vi "VI Properties - Front Panel States.vi"() -> ()   [LabVIEW 2019]
doc: "This VI demonstrates how to programmatically change the state of the front panel window. \n\nThere are six states that are related to the front panel of a VI; Standard, Maximize, Minimize, Hidden, Closed and Invalid. All states are read/write with the exception of Invalid, which is read only. The Standard state sets the VI to its default front panel state. The Maximize state will maximize the VI to full screen size. Minimize state is used to minimize the VI to the task bar. When using the Hidden state, the VI is still in memory, yet the front panel is hidden from view. The Closed state will also hide the front panel of the VI, but the front panel objects of the VI are no longer in memory. Lastly, the Invalid state is returned if an attempt is made to apply a window state at a time when it cannot be applied to the VI."
panel:
  in  "Stop":bool
  in  "Hidden":bool
  in  "Standard":bool
  in  "Minimize":bool
  in  "Maximize":bool
  # "Overview: Programmatically manipulates the state of a VI panel with the Front Panel Window:State property.\nInstructions:\n1. Run the VI. A target VI panel will appear.\n2. Click the various Window States buttons below to manipulate the state of the target VI panel.\n3. Click Stop to stop the VI."
  # "Window States"
  # "Note: This VI is configure to be Modal, meaning that it is always the active and frontmost window. This is done to allow you to investigate the window states of the target VI without having to return to this window. To change the modality setting on a VI, go to File > VI Properties > Window Appearance > Customize > Window Behavior."
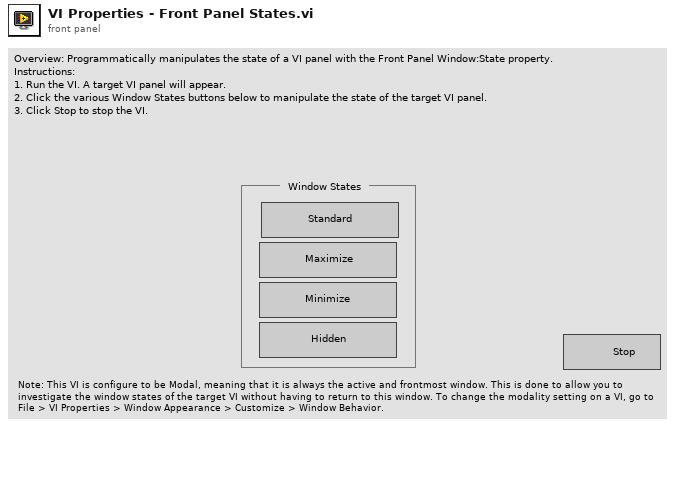
[diagram p1: front panel]
types:
  T1 = enum32{"Invalid", "Standard", "Closed", "Hidden", "Minimized", "Maximized"}
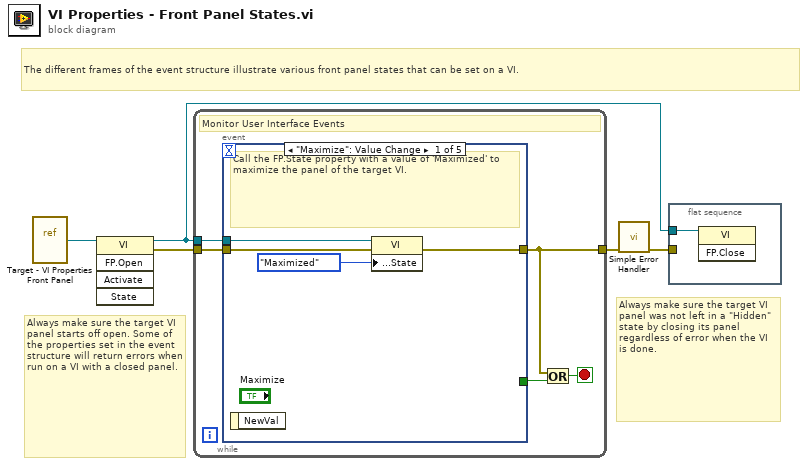
[diagram p0: block diagram]
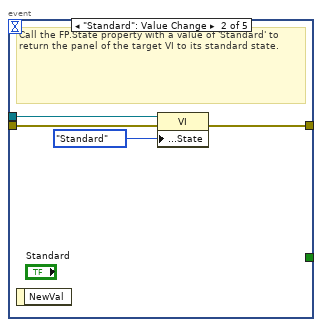
[diagram p2: hidden frame]
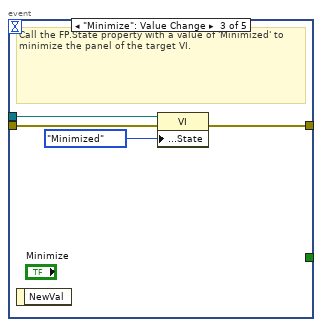
[diagram p3: hidden frame]
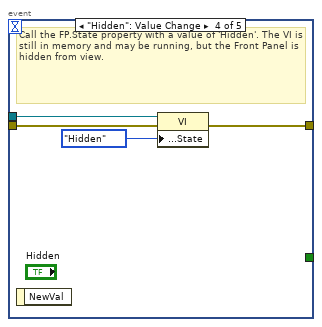
[diagram p4: hidden frame]
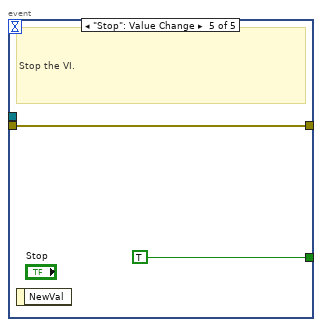
[diagram p5: hidden frame]
diagram:
  # "The different frames of the event structure illustrate various front panel states that can be set on a VI."
  # "Always make sure the target VI panel starts off open. Some of the properties set in the event structure will return errors when run on a VI with a closed panel."
  # "Always make sure the target VI panel was not left in a \"Hidden\" state by closing its panel regardless of error when the VI is done."
  n1 = vi-ref "Target - VI Properties Front Panel.vi"() -> (w3:refnum<vi>)
  n2 = invoke class="VI" method="FP.Open"(reference=w3) -> (reference out=w2:refnum<vi>, error out=w1:errorcluster)  [unwired: 4 in, 3 out]
  n3 = while {
    tunnel: w2 -> [w9]
    tunnel: [w7] -> w5
    tunnel: w1 -> [w6]
    stop <- w8 stop-if-true
    # "Monitor User Interface Events"
    n4 = event shown="[0] \"Maximize\": Value Change" {
      selector: _ -> [_ _ _ _ _]
      dyn-events: _ -> [_ _ _ _ _]
      timeout: _ -> [_ _ _ _ _]
      tunnel: w9 -> [w13 w18 w21 w25 _]
      tunnel: [_ _ _ _ TRUE ("T button?")] -> w10
      tunnel: [w14 w17 w22 w26 w27] -> w7
      tunnel: w6 -> [w11 w15 w19 w23 w27]
      event "Maximize": Value Change {
        # "Call the FP.State property with a value of 'Maximized' to maximize the panel of the target VI."
        n5 = event-data() -> ()  [unwired: 2 out]
        n6 = property class="VI"(reference=w13, error in=w11, "Front Panel Window:State"=T1."Maximized") -> (error out=w14:errorcluster)  [unwired: 1 out]
      }
      event "Standard": Value Change {
        # "Call the FP.State property with a value of 'Standard' to return the panel of the target VI to its standard state."
        n7 = event-data() -> ()  [unwired: 2 out]
        n8 = property class="VI"(reference=w18, error in=w15, "Front Panel Window:State"=T1."Standard") -> (error out=w17:errorcluster)  [unwired: 1 out]
      }
      event "Minimize": Value Change {
        # "Call the FP.State property with a value of 'Minimized' to minimize the panel of the target VI."
        n9 = event-data() -> ()  [unwired: 2 out]
        n10 = property class="VI"(reference=w21, error in=w19, "Front Panel Window:State"=T1."Minimized") -> (error out=w22:errorcluster)  [unwired: 1 out]
      }
      event "Hidden": Value Change {
        # "Call the FP.State property with a value of 'Hidden'. The VI is still in memory and may be running, but the Front Panel is hidden from view."
        n11 = event-data() -> ()  [unwired: 2 out]
        n12 = property class="VI"(reference=w25, error in=w23, "Front Panel Window:State"=T1."Hidden") -> (error out=w26:errorcluster)  [unwired: 1 out]
      }
      event "Stop": Value Change {
        # "Stop the VI."
        n13 = event-data() -> ()  [unwired: 2 out]
      }
    }
    n14 = Or(x=w7, y=w10) -> (x .or. y?=w8:bool)
  }
  n15 = call <vilib>:"Simple Error Handler.vi"("error in (no error)"=w5) -> ("error out"=w4:errorcluster)  [unwired: 1 in, 7 out]
  n16 = flat-sequence {
    tunnel: w4 -> [_]
    tunnel: w2 -> [w29]
    frame #0 {
      n17 = invoke class="VI" method="FP.Close"(reference=w29) -> ()  [unwired: 2 in, 3 out]
    }
  }
